vi "GetSingleFrame.vi"() -> ()   [LabVIEW 2015]
uses:
  <vilib>/addons/h5labview2/dataset/H5Dread.llb/H5Dread.xnode
  <vilib>/addons/h5labview2/space/H5S.lvlib
  <vilib>/addons/h5labview2/base/H5Equery.vi
  <vilib>/addons/h5labview2/base/lib_path.vi
  <vilib>/addons/h5labview2/base/hid_t.ctl
panel:
  in  "y pixels":dbl
  in  "X pixels":dbl
  in  "error in (no error)":errorcluster
  in  "ref in":T1 format="%.0x"
  out "dims":u32[](array[numeric])
  out "Data out":u16[](array[numeric])
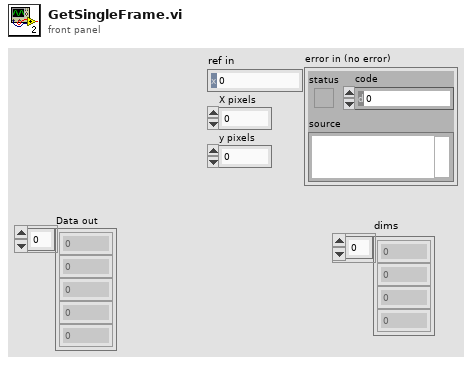
[diagram p1: front panel]
types:
  T1 = typedef "hid_t.ctl" = i32
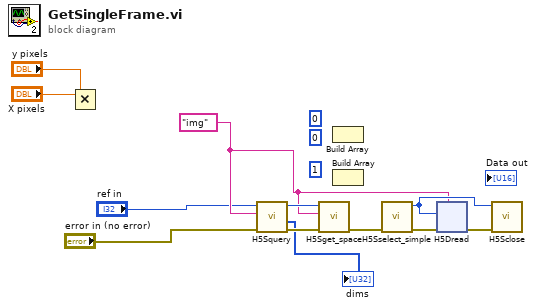
[diagram p0: block diagram]
diagram:
  (unwired) 0 ("element")
  (unwired) 0
  (unwired) 1 ("element")
  w6 = "img" ("Combo Box")
  n1 = Multiply(x="X pixels", y="y pixels") -> ()  [unwired: 1 out]
  n2 = call <vilib>:"H5Squery.vi"("error in (no error)"="error in (no error)", "obj"=w6, "ref in"="ref in") -> ("error out"=w8:errorcluster, "dims"=→"dims":u32[], "ref out"=w9:T1)  [unwired: 5 in, 1 out]
  n3 = call <vilib>:"H5Sget_space.vi"("error in (no error)"=w8, "obj"=w6, "ref in"=w9) -> ("error out"=w7:errorcluster)  [unwired: 7 in, 1 out]
  n4 = Build Array() -> ()  [unwired: 2 in, 1 out]
  n5 = Build Array() -> ()  [unwired: 2 in, 1 out]
  n6 = call <vilib>:"H5Sselect_simple.vi"("error in (no error)"=w7) -> ("error out"=w12:errorcluster, "space out"=w10:T1)  [unwired: 9 in]
  n7 = xnode "H5Dread"("dataset name (this)"=w6, "error in (no error)"=w12, "file space"=w10) -> ("error out"=w11:errorcluster)  [unwired: 3 in, 3 out]
  n8 = call <vilib>:"H5Sclose.vi"("error in (no error)"=w11, "space in"=w10) -> ()  [unwired: 9 in, 1 out]
